vi "Convert 2 DBL Arrays to Strings.vi"(7 "Y Values Label":string="Strain Gauge (Volts)", 10 "X Values (Seconds)":dbl[](array[numeric]), 11 "Y Values (Voltage)":dbl[](array[numeric])) -> (2 "DataSet Rows":string[](array[string]))   [LabVIEW 2021]
doc: "Converts dataset into strings, and prepends a column header."
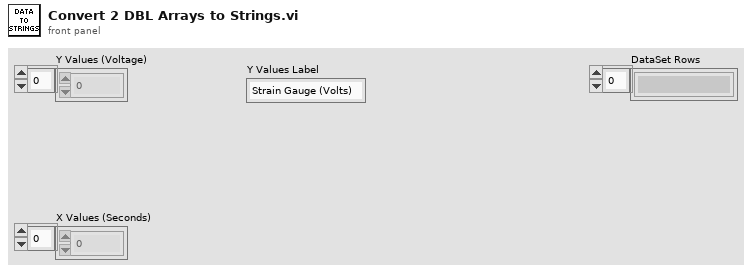
[diagram p1: front panel]
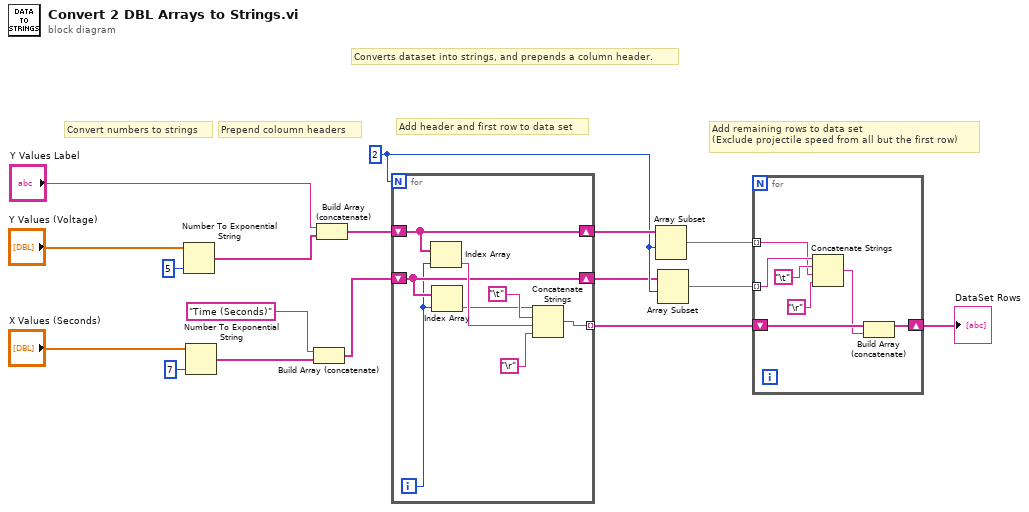
[diagram p0: block diagram]
diagram:
  w6 = 2
  # "Add remaining rows to data set\n(Exclude projectile speed from all but the first row)"
  # "Add header and first row to data set"
  # "Convert numbers to strings"
  # "Prepend coloumn headers"
  # "Converts dataset into strings, and prepends a column header."
  n1 = Number To Exponential String(number="Y Values (Voltage)", precision (6)=i16 5) -> (E-format string=w13:string[])  [unwired: 2 in]
  n2 = Number To Exponential String(number="X Values (Seconds)", precision (6)=i16 7) -> (E-format string=w11:string[])  [unwired: 2 in]
  n3 = Build Array (concatenate)("Time (Seconds)", w11) -> (w10:string[])
  n4 = Build Array (concatenate)("Y Values Label", w13) -> (w9:string[])
  n5 = for {
    N: w6 -> [_]
    tunnel: [w24] -> w8 mode=indexing
    shift-right: [w23] -> w7
    shift-left: w9 -> [w23]
    shift-right: [w21] -> w5
    shift-left: w10 -> [w21]
    i -> [w19]
    n6 = Index Array(array=w23, index=w19) -> (element=w22:string)
    n7 = Index Array(array=w21, index=w19) -> (element=w20:string)
    n8 = Concatenate Strings(w20, "\t", w22, "\r") -> (w24:string)
  }
  n9 = Array Subset(array=w7, index=w6) -> (w3:string[])  [unwired: 1 in]
  n10 = Array Subset(array=w5, index=w6) -> (w4:string[])  [unwired: 1 in]
  n11 = for {
    tunnel: w4 -> [w31] mode=indexing
    tunnel: w3 -> [w29] mode=indexing
    shift-right: [w27] -> w2
    shift-left: w8 -> [w32]
    n12 = Concatenate Strings(w31, "\t", w29, "\r") -> (w28:string)
    n13 = Build Array (concatenate)(w32, w28) -> (w27:string[])
  }
  "DataSet Rows" <- w2
